vi "ChemTrac read all.vi"(4 "State":i16=-1, 5 "Time":dbl format="%.2f", 6 "Sensor Values":dbl[](array[numeric]), 7 "Set Points":dbl[](array[numeric])=[1.0, 3.0, 1.0]) -> (0 "required data":T6={"Set Point names"=["data interval (s)", "device ID"], "required number of setpoints"=2, "required number of sensors"=0, "Sensor names"=[]}, 3 "output value":dbl)   [LabVIEW 2019]
uses:
  modbusrtu/MB ID-Address.ctl
  modbusrtu/SerialParameters.ctl
  modbusrtu/MB status.ctl
  modbusrtu/ProCoDA MB Request.ctl
  modbusrtu/Read Write.ctl
  modbusrtu/MB cmd buffer.ctl
panel:
  in  "MB status":T1 {"MB update(s)" format="%.2g"; "ProCoDA Request"."PC update (s)" format="%.2f"; "ProCoDA Request"."# registers" min=1}
  in  "MB ID-Address":T4
  # "Input Registers (Read Only)\nModbus Map: HydroAct 4 (75FC:4543:F24F:4856)\nAddress Size Type Device Description Ref.\n0 2 FLOAT UV-254 1.1 Official Value - UVA\n2 2 FLOAT UV-254 1.1 Official Value - UVT\n4 2 FLOAT UV-254 1.1 Official Value - Compensated UVA\n6 2 FLOAT UV-254 1.1 Official Value - COD\n8 2 FLOAT UV-254 1.1 Official Value - TOC\n10 2 FLOAT Particle Counter 1.2 Official Value - Cell\n12 2 FLOAT Particle Counter 1.2 Official Value - Laser\n14 2 FLOAT Particle Counter 1.2 Official Value - Total Counts\n16 2 FLOAT Particle Counter 1.2 Official Value - Counts Bin 1\n18 2 FLOAT Particle Counter 1.2 Official Value - Counts Bin 2\n20 2 FLOAT Particle Counter 1.2 Official Value - Counts Bin 3\n22 2 FLOAT Particle Counter 1.2 Official Value - Counts Bin 4\n24 2 FLOAT Particle Counter 1.2 Official Value - Counts Bin 5\n26 2 FLOAT Particle Counter 1.2 Official Value - Counts Bin 6\n28 2 FLOAT Particle Counter 1.2 Official Value - Total PPB\n30 2 FLOAT Particle Counter 1.2 Official Value - PPB Bin 1\n32 2 FLOAT Particle Counter 1.2 Official Value - PPB Bin 2\n34 2 FLOAT Particle Counter 1.2 Official Value - PPB Bin 3\n36 2 FLOAT Particle Counter 1.2 Official Value - PPB Bin 4\n38 2 FLOAT Particle Counter 1.2 Official Value - PPB Bin 5\n40 2 FLOAT Particle Counter 1.2 Official Value - PPB Bin 6\n42 2 FLOAT Particle Counter 1.3 Official Value - Cell\n44 2 FLOAT Particle Counter 1.3 Official Value - Laser\n46 2 FLOAT Particle Counter 1.3 Official Value - Total Counts\n48 2 FLOAT Particle Counter 1.3 Official Value - Counts Bin 1\n50 2 FLOAT Particle Counter 1.3 Official Value - Counts Bin 2\n52 2 FLOAT Particle Counter 1.3 Official Value - Counts Bin 3\n54 2 FLOAT Particle Counter 1.3 Official Value - Counts Bin 4\n56 2 FLOAT Particle Counter 1.3 Official Value - Counts Bin 5\n58 2 FLOAT Particle Counter 1.3 Official Value - Counts Bin 6\n60 2 FLOAT Particle Counter 1.3 Official Value - Total PPB\n62 2 FLOAT Particle Counter 1.3 Official Value - PPB Bin 1\n64 2 FLOAT Particle Counter 1.3 Official Value - PPB Bin 2\n66 2 FLOAT Particle Counter 1.3 Official Value - PPB Bin 3\n68 2 FLOAT Particle Counter 1.3 Official Value - PPB Bin 4\n70 2 FLOAT Particle Counter 1.3 Official Value - PPB Bin 5\n72 2 FLOAT Particle Counter 1.3 Official Value - PPB Bin 6"
  # "Enter the correct information for this control code in the required data structure below. Then make the current value default by right clicking on the border of the data structure. Select \"data operations\" and then select \"make current value default\". These values will be displayed by process controller."
  # "HydroACT has even parity by default."
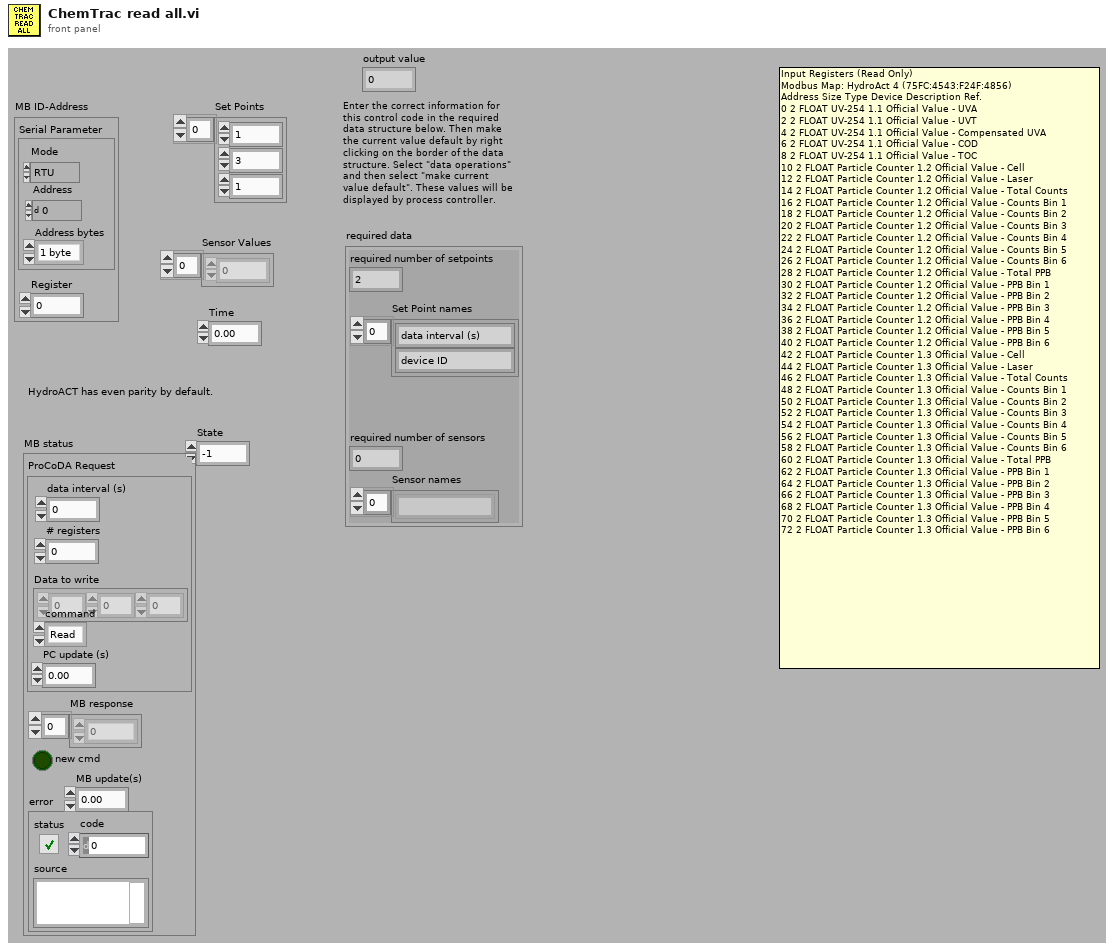
[diagram p1: front panel]
types:
  T1 = typedef "MB status.ctl" = cluster{"ProCoDA Request":T2, "MB response":dbl[], "new cmd":bool, "error":errorcluster, "MB update(s)":dbl}
  T2 = typedef "ProCoDA MB Request.ctl" = cluster{"# registers":u8, "Data to write":u16[], "data interval (s)":dbl, "command":T3, "PC update (s)":dbl}
  T3 = typedef "Read Write.ctl" = enum16{"Read", "Write"}
  T4 = typedef "MB ID-Address.ctl" = cluster{"Serial Parameter":T5, "Register":u16}
  T5 = typedef "SerialParameters.ctl" = cluster{"Mode":enum16{"RTU", "ASCII"}, "Address":u16, "Address bytes":enum16{"1 byte", "2 bytes"}}
  T6 = cluster{"Set Point names":string[], "required number of setpoints":u8, "required number of sensors":u8, "Sensor names":string[]}
  T7 = cluster{"Set Points[0]":dbl, "Set Points[1]":dbl}
  T8 = typedef "MB cmd buffer.ctl" = enum16{"ProCoDA", "MB succeed", "MB error", "MB Next Task", "ProCoDA read 1", "Commands pending"}
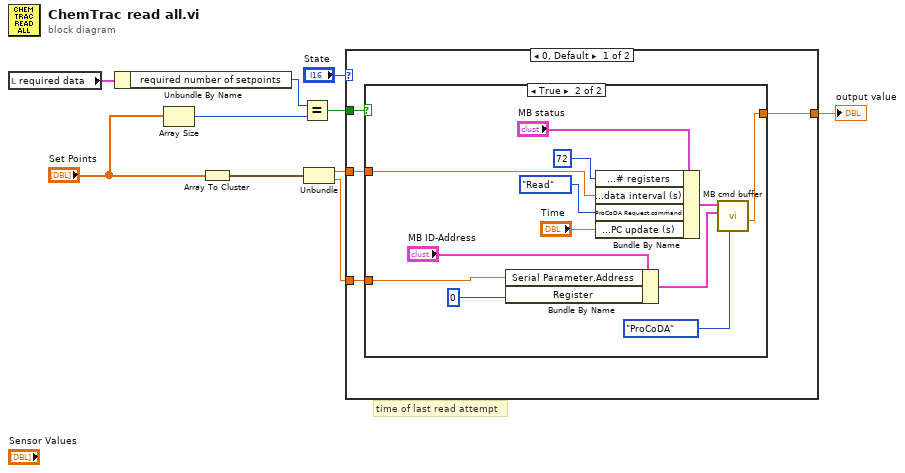
[diagram p0: block diagram]
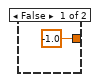
[diagram p2: hidden frame]
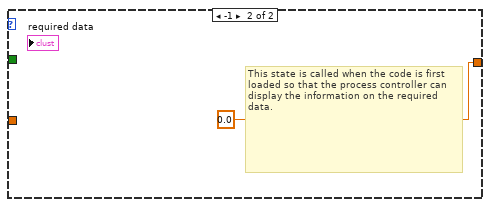
[diagram p3: hidden frame]
diagram:
  # "time of last read attempt"
  n1 = local read "required data"() -> (w4:T6)
  n2 = Unbundle By Name(w4) -> ("required number of setpoints"=w3:u8)
  n3 = Array Size(array="Set Points") -> (size(s)=w6:i32)
  n4 = Array To Cluster(array="Set Points") -> (cluster=w8:T7)
  n5 = Equal?(x=w3, y=w6) -> (x = y?=w5:bool)
  n6 = Unbundle(w8) -> ("Set Points[0]"=w2:dbl, "Set Points[1]"=w1:dbl)
  n7 = case shown="0, Default" "State" {
    tunnel: [w11 0.0 ("fraction on")] -> w9
    tunnel: w5 -> [w14 _]
    tunnel: w2 -> [w13 _]
    tunnel: w1 -> [w12 _]
    frame 0, Default {
      n8 = case shown="True" w14 {
        tunnel: [-1.0 ("fraction on") w18] -> w11
        tunnel: w13 -> [_ w23]
        tunnel: w12 -> [_ w19]
        frame False {
        }
        frame True {
          n9 = Bundle By Name(cluster="MB ID-Address", "Serial Parameter.Address"=w19, "Register"=u8 0 ("MB ID-Address.Address")) -> (w16:T4)
          n10 = Bundle By Name(cluster="MB status", "ProCoDA Request.# registers"=u8 72 ("# registers"), "ProCoDA Request.data interval (s)"=w23, "ProCoDA Request.command"=Read_Write."Read" ("command"), "ProCoDA Request.PC update (s)"="Time") -> (w25:T1)
          n11 = call "MB cmd buffer.vi"("MB cmd buffer"=MB_cmd_buffer."ProCoDA", "MB ID-Address in"=w16, "MB status in"=w25) -> ("output value"=w18:dbl)  [unwired: 2 in, 6 out]
        }
      }
    }
    frame -1 {
      # "This state is called when the code is first loaded so that the process controller can display the information on the required data."
    }
  }
  "output value" <- w9
